vi "test Loopback_Acyclic_SelectiveTrigger.vi"(8 "error in":errorcluster, 11 "TestCase in":refnum<class "SingleCore.lvclass">) -> (0 "error out":errorcluster, 3 "TestCase out":refnum<class "SingleCore.lvclass">)   [LabVIEW 2020, in "SingleCore.lvclass"]
uses:
  SingleCore.lvclass
  C:/Git/niveristand-custom-device-testing-tools/VeriStandTestCase/VeriStandTestCase.lvclass
  4b06c685-66bb-4135-9ad1-d89a50a95502.vi
  <vilib>/numeric/Random Number (Range) I64.vi
  <vilib>/numeric/sub_Random U32.vi
  <vilib>/NI VeriStand/Execution/Workspace/NI VeriStand - Set Multiple Channel Values.vi
  <vilib>/addons/_JKI Toolkits/VI Tester/TestCase.llb/TestCase.lvclass
  <vilib>/NI VeriStand/Execution/Workspace/NI_VS Workspace ExecutionAPI.lvlib
  C:/Program Files (x86)/National Instruments/LabVIEW 2020/vi.lib/addons/_JKI Toolkits/VI Tester/TestCase.llb/TestCase.lvclass
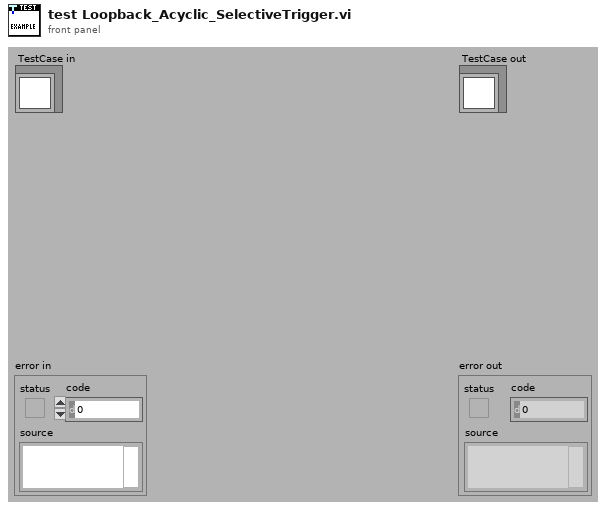
[diagram p1: front panel]
types:
  T1 = typedef "NI_VS Workspace ExecutionAPI.lvlib/WorkspaceAPI.ctl" = refnum<k24>
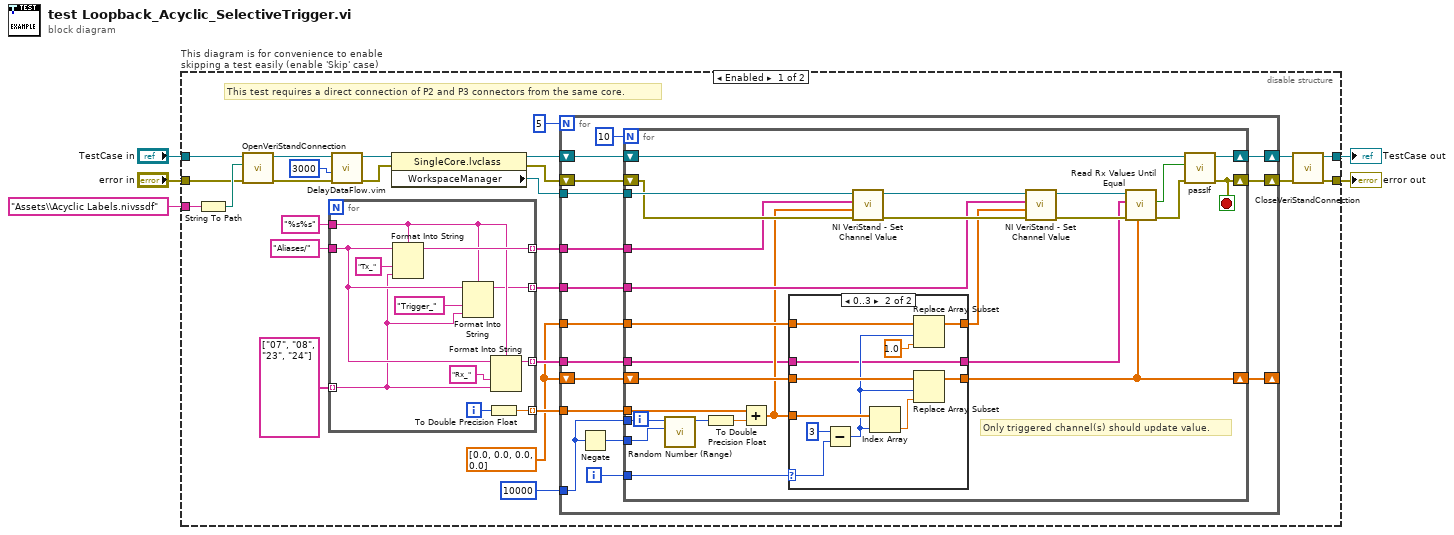
[diagram p0: block diagram]
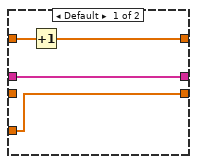
[diagram p2: hidden frame]
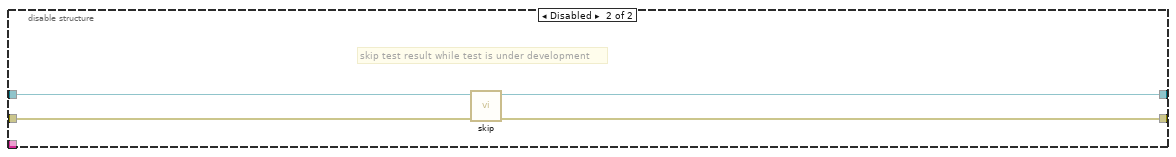
[diagram p3: hidden frame]
diagram:
  n1 = disable-structure "This diagram is for convenience to enable skipping a test easily (enable 'Skip' case)" shown="Enabled" {
    disable-tunnel: "TestCase in" -> [w25 w102]
    disable-tunnel: [w22 w100] -> w2
    disable-tunnel: [w21 w101] -> w4
    disable-tunnel: "error in" -> [w24 w99]
    disable-tunnel: "Assets\\Acyclic Labels.nivssdf" ("Channel") -> [w23 _]
    frame Enabled {
      w6 = dbl[] [0.0, 0.0, 0.0, 0.0] ("Values")
      # "This test requires a direct connection of P2 and P3 connectors from the same core."
      n2 = String To Path(string=w23) -> (path=w26:path)
      n3 = call-dynamic "OpenVeriStandConnection.vi"("error in (no error)"=w24, "System Definition File"=w26, "VeriStand Test Case in"=w25) -> ("error out"=w28:errorcluster, "VeriStand Test Case out"=w30:refnum<class "SingleCore.lvclass">)  [unwired: 6 in, 1 out]
      n4 = for {
        tunnel: [w98] -> w18 mode=indexing
        tunnel: [w93] -> w15 mode=indexing
        tunnel: [w97] -> w20 mode=indexing
        tunnel: "Aliases/" ("Channel") -> [w91]
        tunnel: string[] ["07", "08", "23", "24"] -> [w89] mode=indexing
        tunnel: "%s%s" ("format string") -> [w92]
        tunnel: [w88] -> w7 mode=indexing
        i -> [w96]
        n5 = Format Into String(format string=w92, initial string=w91, "Tx_" ("input 1"), w89) -> (resulting string=w98:string)  [unwired: 1 in, 1 out]
        n6 = Format Into String(format string=w92, initial string=w91, "Trigger_" ("input 1"), w89) -> (resulting string=w88:string)  [unwired: 1 in, 1 out]
        n7 = To Double Precision Float(number=w96) -> (double precision float=w97:dbl)
        n8 = Format Into String(format string=w92, initial string=w91, "Rx_" ("input 1"), w89) -> (resulting string=w93:string)  [unwired: 1 in, 1 out]
      }
      n9 = call "DelayDataFlow.vim"("value in"=w28, "milliseconds to wait"=u32 3000) -> ("value out"=w27:errorcluster)  [unwired: 2 in, 1 out]
      n10 = property class="SingleCore.lvclass"(reference=w30, error in=w27) -> (reference out=w14:refnum<class "SingleCore.lvclass">, error out=w16:errorcluster, "WorkspaceManager"=w17:T1)
      n11 = for {
        N: 5 -> [_]
        tunnel: w20 -> [w46]
        tunnel: i64 10000 ("upper bound (100)") -> [w45]
        tunnel: w18 -> [w44]
        tunnel: w17 -> [w43]
        tunnel: w15 -> [w41]
        shift-right: [w38] -> w12
        shift-left: w16 -> [w42]
        shift-right: [w39] -> w13
        shift-left: w14 -> [w40]
        tunnel: w7 -> [w36]
        shift-right: [w33] -> _
        shift-left: w6 -> [w35]
        tunnel: w6 -> [w34]
        i -> [w37]
        n12 = Negate(x=w45) -> (-x=w32:i64)
        n13 = for {
          N: 10 -> [_]
          tunnel: w46 -> [w71]
          tunnel: w45 -> [w70]
          tunnel: w32 -> [w69]
          tunnel: w44 -> [w60]
          tunnel: w43 -> [w62]
          tunnel: w41 -> [w47]
          shift-right: [w68] -> w39
          shift-left: w40 -> [w59]
          shift-right: [w67] -> w38
          shift-left: w42 -> [w61]
          tunnel: w37 -> [w57]
          tunnel: w36 -> [w58]
          shift-right: [w49] -> w33
          shift-left: w35 -> [w51]
          tunnel: w34 -> [w52]
          stop <- w67 stop-if-true
          # "Only triggered channel(s) should update value."
          n14 = call-poly <vilib>:"Random Number (Range).vi"("lower bound (-100)"=w69, "upper bound (100)"=w70) -> ("number"=w72:i64)  [unwired: 9 in]
          n15 = To Double Precision Float(number=w72) -> (double precision float=w55:dbl)
          n16 = Add(x=w71, y=w55) -> (x+y=w50:dbl[])
          n17 = case shown="0..3" w57 {
            selector: w57 -> [_ w87]
            tunnel: [w75 w84] -> w56
            tunnel: w52 -> [w76 w83]
            tunnel: w51 -> [_ w82]
            tunnel: w50 -> [w74 w81]
            tunnel: [w74 w79] -> w49
            tunnel: [w73 w77] -> w48
            tunnel: w47 -> [w73 w77]
            frame Default {
              n18 = Increment(x=w76) -> (x+1=w75:dbl[])
            }
            frame 0..3 {
              n19 = Subtract(x=3, y=w87) -> (x-y=w78:i32)
              n20 = Index Array(array=w81, index=w78) -> (element=w80:dbl)
              n21 = Replace Array Subset(array=w83, new element=1.0 ("new element/subarray"), index=w78) -> (w84:dbl[])
              n22 = Replace Array Subset(array=w82, new element=w80, index=w78) -> (w79:dbl[])
            }
          }
          n23 = call-poly <vilib>:"NI VeriStand - Set Channel Value.vi"("error in (no error)"=w61, "Values"=w50, "Channels"=w60, "WorkspaceManager in"=w62) -> ("error out"=w63:errorcluster, "WorkspaceManager out"=w66:T1)  [unwired: 6 in]
          n24 = call-poly <vilib>:"NI VeriStand - Set Channel Value.vi"("error in (no error)"=w63, "Values"=w56, "Channels"=w58, "WorkspaceManager in"=w66) -> ("error out"=w64:errorcluster, "WorkspaceManager out"=w65:T1)  [unwired: 6 in]
          n25 = call "Read Rx Values Until Equal.vi"("expected values"=w49, "error in"=w64, "Rx aliases"=w48, "workspace manager in"=w65) -> ("error out"=w53:errorcluster, "values equal expected"=w54:bool)  [unwired: 5 in, 1 out]
          n26 = call-dynamic "passIf.vi"("error in (no error)"=w53, "pass"=w54, "TestCase in"=w59) -> ("error out"=w67:errorcluster, "TestCase out"=w68:refnum<class "SingleCore.lvclass">)  [unwired: 7 in]
        }
      }
      n27 = call-dynamic "CloseVeriStandConnection.vi"("error in (no error)"=w12, "VeriStand Test Case in"=w13) -> ("error out"=w21:errorcluster, "VeriStand Test Case out"=w22:refnum<class "SingleCore.lvclass">)  [unwired: 8 in]
    }
    frame Disabled {
      # "skip test result while test is under development"
      n28 = call <vilib>:"skip.vi"("error in (no error)"=w99, "TestCase in"=w102) -> ("error out"=w101:errorcluster, "TestCase out"=w100:refnum<class "SingleCore.lvclass">)  [unwired: 8 in]
    }
  }
  "error out" <- w4
  "TestCase out" <- w2
